vi "Pic Overlay o Point.vi"(8 "error in (no error)":errorcluster, 10 "Picture in":picture, 11 "LF2R IDE in":refnum<class "Main Panel.lvclass">) -> (0 "error out":errorcluster, 2 "Picture out":picture, 3 "LF2R IDE out":refnum<class "Main Panel.lvclass">)   [LabVIEW 2018, in "Main Panel.lvlib" / "Main Panel.lvclass"]
uses:
  Main Panel.lvclass
  Main Panel.lvclass/Main Panel.ctl
  Picture Process/Picture Process.lvclass
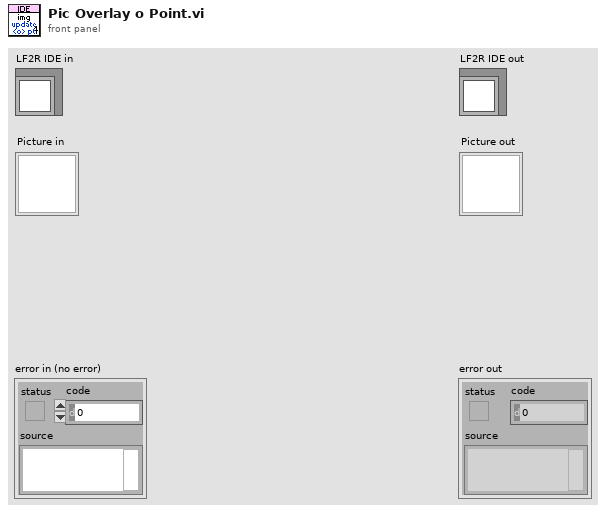
[diagram p1: front panel]
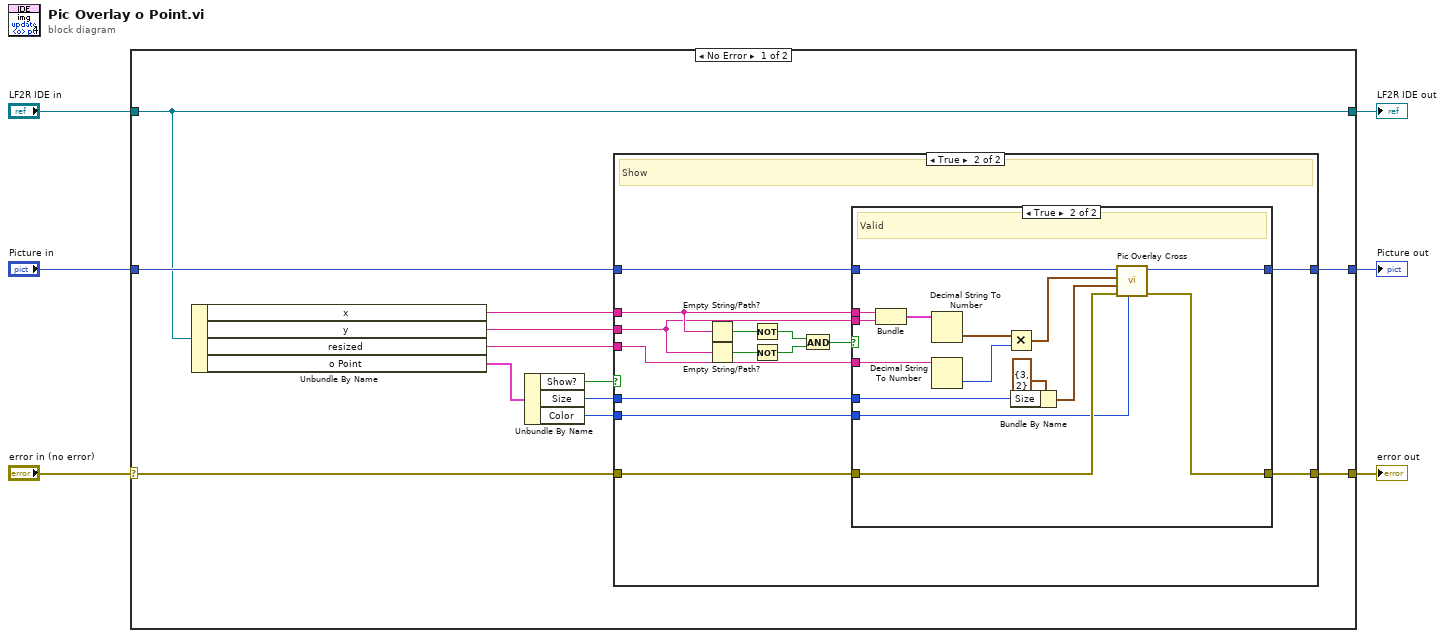
[diagram p0: block diagram]
diagram:
  n1 = case shown="No Error" "error in (no error)" {
    selector: "error in (no error)" -> [w16 w54]
    tunnel: [w18 w54] -> w5
    tunnel: [w8 w53] -> w3
    tunnel: "LF2R IDE in" -> [w8 w53]
    tunnel: "Picture in" -> [w9 w52]
    tunnel: [w7 w52] -> w1
    frame No Error {
      n2 = Unbundle By Name(w8) -> ("x"=w15:string, "y"=w14:string, "resized"=w17:string, "o Point"=w13:cluster{"Size":i32, "Color":u32, "Show?":bool})
      n3 = Unbundle By Name(w13) -> ("Show?"=w12:bool, "Size"=w11:i32, "Color"=w10:u32)
      n4 = case shown="True" w12 {
        tunnel: [w20 w34] -> w18
        tunnel: w17 -> [_ w33]
        tunnel: w16 -> [w20 w32]
        tunnel: w15 -> [_ w31]
        tunnel: w14 -> [_ w30]
        tunnel: w11 -> [_ w24]
        tunnel: w10 -> [_ w23]
        tunnel: w9 -> [w19 w22]
        tunnel: [w19 w21] -> w7
        frame False {
          # "Skip"
        }
        frame True {
          # "Show"
          n5 = Empty String/Path?(string/path=w31) -> (empty?=w29:bool)
          n6 = Empty String/Path?(string/path=w30) -> (empty?=w28:bool)
          n7 = Not(x=w29) -> (.not. x?=w27:bool)
          n8 = Not(x=w28) -> (.not. x?=w26:bool)
          n9 = And(x=w27, y=w26) -> (x .and. y?=w25:bool)
          n10 = case shown="True" w25 {
            tunnel: [w36 w38] -> w34
            tunnel: w33 -> [_ w51]
            tunnel: w32 -> [w36 w40]
            tunnel: w31 -> [_ w48]
            tunnel: w30 -> [_ w47]
            tunnel: w24 -> [_ w42]
            tunnel: w23 -> [_ w39]
            tunnel: w22 -> [w35 w45]
            tunnel: [w35 w37] -> w21
            frame False {
              # "Invalid"
            }
            frame True {
              # "Valid"
              n11 = Bundle("x"=w48, "y"=w47) -> (w46:cluster{"x":string, "y":string})  [unwired: 1 in]
              n12 = Decimal String To Number(string=w46) -> (number=w50:cluster{"x":i32, "y":i32})  [unwired: 2 in, 1 out]
              n13 = Decimal String To Number(string=w51) -> (number=w49:i32)  [unwired: 2 in, 1 out]
              n14 = Multiply(x=w50, y=w49) -> (x*y=w44:cluster{"x":i32, "y":i32})
              n15 = Bundle By Name(cluster=cluster{"Size":i32, "Width":u16} {"Size"=3, "Width"=2} ("Line"), "Size"=w42) -> (w41:cluster{"Size":i32, "Width":u16})
              n16 = call "Pic Overlay Cross.vi"("Color"=w39, "error in (no error)"=w40, "Line"=w41, "Position"=w44, "Picture in"=w45) -> ("error out"=w38:errorcluster, "Picture out"=w37:picture)  [unwired: 5 in]
            }
          }
        }
      }
    }
    frame Error {
    }
  }
  "error out" <- w5
  "LF2R IDE out" <- w3
  "Picture out" <- w1
